vi "PQgetTable.vi"(8 "error in":errorcluster, 10 "query":string, 11 "conn":u32) -> (0 "error out":errorcluster, 1 "Data":string[][](array[string]), 3 "conn_out":u32, 4 "PQnFields":i32, 6 "PQnTuples":i32)   [LabVIEW 2019, in "libpqutility.lvlib"]
uses:
  libpqutility.lvlib
  libpqlv/libpqlv.lvlib
panel:
  out "PQsendQuery":i32
  out "PQresultStatus":T1(ring)
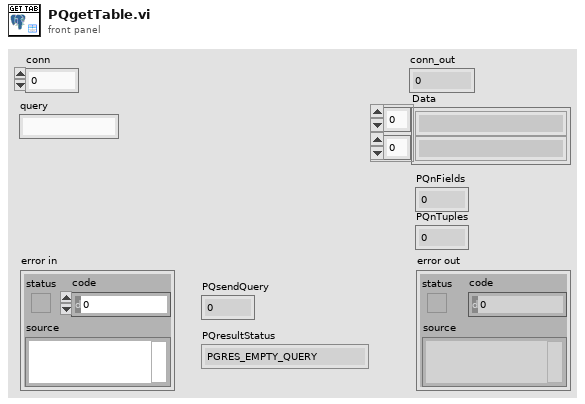
[diagram p1: front panel]
types:
  T1 = enum32{"PGRES_EMPTY_QUERY", "PGRES_COMMAND_OK", "PGRES_TUPLES_OK", "PGRES_COPY_OUT", "PGRES_COPY_IN", "PGRES_BAD_RESPONSE", "PGRES_NONFATAL_ERROR", "PGRES_FATAL_ERROR"}
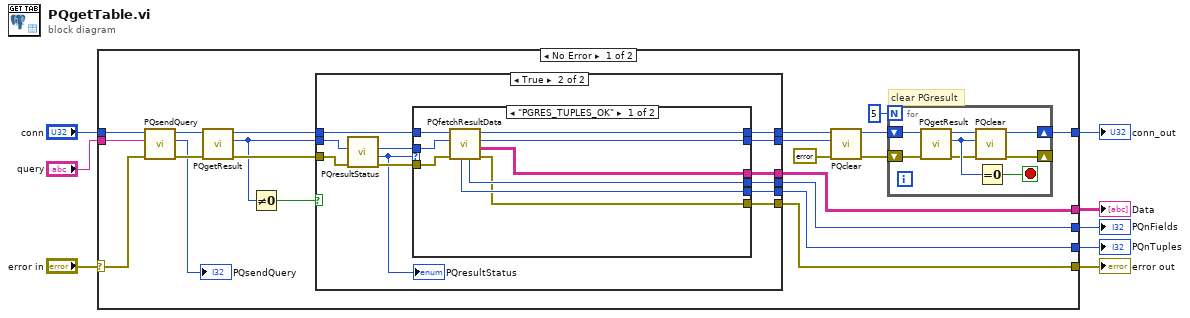
[diagram p0: block diagram]
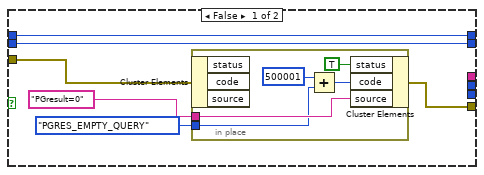
[diagram p2: hidden frame]
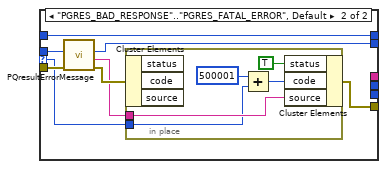
[diagram p3: hidden frame]
diagram:
  n1 = case shown="No Error" "error in" {
    selector: "error in" -> [w22 w84]
    tunnel: "conn" -> [w23 w83]
    tunnel: [w24 w84] -> w7
    tunnel: [w11 w83] -> w5
    tunnel: [w21 _] -> w4
    tunnel: "query" -> [w18 _]
    tunnel: [w17 _] -> w2
    tunnel: [w16 _] -> w1
    frame No Error {
      # "clear PGresult"
      n2 = call "PQsendQuery.vi"("error in (no error)"=w22, "query"=w18, "conn"=w23) -> ("error out"=w29:errorcluster, "PQsendQuery"=→"PQsendQuery":i32, "conn_out"=w20:u32)  [unwired: 6 in]
      n3 = call "PQgetResult.vi"("error in (no error)"=w29, "conn"=w20) -> ("error out"=w28:errorcluster, "PGresult"=w27:u32, "conn_out"=w19:u32)  [unwired: 7 in]
      n4 = Not Equal To 0?(x=w27) -> (x != 0?=w26:bool)
      n5 = case shown="True" w26 {
        tunnel: w28 -> [w39 w60]
        tunnel: w19 -> [w42 w59]
        tunnel: [_ w57] -> w21
        tunnel: [_ w56] -> w17
        tunnel: [w38 w55] -> w24
        tunnel: w27 -> [w43 w53]
        tunnel: [_ w54] -> w16
        tunnel: [w43 w51] -> w9
        tunnel: [w42 w49] -> w10
        frame False {
          n6 = in-place {
            in-place-border: "PGresult=0" ("source") -> [w48]
            in-place-border: T1."PGRES_EMPTY_QUERY" ("PQresultStatus") -> [w45]
            n7 = in-place-cluster #1(w39) -> ()  [unwired: 3 out]
            n8 = Add(x=u32 500001, y=w45) -> (x+y=w44:u32)
            n9 = in-place-cluster #1("status"=TRUE, "code"=w44, "source"=w48) -> (w38:errorcluster)
          }
        }
        frame True {
          n10 = call "PQresultStatus.vi"("error in (no error)"=w60, "res"=w53) -> ("error out"=w58:errorcluster, "PQresultStatus"=w52:T1, "res out"=w50:u32)  [unwired: 7 in]
          "PQresultStatus" <- w52
          n11 = case shown="\"PGRES_TUPLES_OK\"" w52 {
            selector: w52 -> [_ w71]
            tunnel: w50 -> [w67 w75]
            tunnel: [w62 _] -> w56
            tunnel: w58 -> [w64 w77]
            tunnel: w59 -> [w68 w76]
            tunnel: [w65 _] -> w57
            tunnel: [w61 w70] -> w55
            tunnel: [w63 _] -> w54
            tunnel: [w66 w74] -> w51
            tunnel: [w69 w76] -> w49
            frame "PGRES_TUPLES_OK" {
              n12 = call "PQfetchResultData.vi"("error in"=w64, "res"=w67, "conn"=w68) -> ("error out"=w61:errorcluster, "Data"=w65:string[][], "res_out"=w66:u32, "conn_out"=w69:u32, "PQnFields"=w62:i32, "PQnTuples"=w63:i32)  [unwired: 3 in]
            }
            frame "PGRES_BAD_RESPONSE".."PGRES_FATAL_ERROR", Default {
              n13 = call "PQresultErrorMessage.vi"("error in (no error)"=w77, "res"=w75) -> ("error out"=w73:errorcluster, "PQresultErrorMessage"=w72:string, "res out"=w74:u32)  [unwired: 7 in]
              n14 = in-place {
                in-place-border: w72 -> [w82]
                in-place-border: w71 -> [w79]
                n15 = in-place-cluster #2(w73) -> ()  [unwired: 3 out]
                n16 = Add(x=u32 500001, y=w79) -> (x+y=w78:u32)
                n17 = in-place-cluster #2("status"=TRUE, "code"=w78, "source"=w82) -> (w70:errorcluster)
              }
            }
          }
        }
      }
      n18 = call "PQclear.vi"("error in (no error)"=errorcluster {"status"=FALSE, "code"=0, "source"=""}, "res"=w9, "conn"=w10) -> ("error out"=w13:errorcluster, "conn_out"=w14:u32)  [unwired: 7 in]
      n19 = for {
        N: 5 -> [_]
        shift-right: [w33] -> w11
        shift-left: w14 -> [w34]
        shift-right: [w30] -> _
        shift-left: w13 -> [w32]
        stop <- w36 stop-if-true
        n20 = call "PQgetResult.vi"("error in (no error)"=w32, "conn"=w34) -> ("error out"=w31:errorcluster, "PGresult"=w35:u32, "conn_out"=w37:u32)  [unwired: 7 in]
        n21 = call "PQclear.vi"("error in (no error)"=w31, "res"=w35, "conn"=w37) -> ("error out"=w30:errorcluster, "conn_out"=w33:u32)  [unwired: 7 in]
        n22 = Equal To 0?(x=w35) -> (x = 0?=w36:bool)
      }
    }
    frame Error {
    }
  }
  "conn_out" <- w5
  "error out" <- w7
  "Data" <- w4
  "PQnFields" <- w2
  "PQnTuples" <- w1
